vi "Login.vi"(8 "error in (no error)":errorcluster, 11 "reference in":refnum<class "Test_Base.lvclass">) -> (0 "error out":errorcluster, 1 "cancelled":bool, 2 "valid":bool, 3 "reference in":refnum<class "Test_Base.lvclass">)   [LabVIEW 2022 SP3, in "Test_Base.lvlib" / "Test_Base.lvclass"]
uses:
  Test_Base.lvclass
  Components/MES_Base.lvlibp/MES_Base.lvclass
  Components/TestView_Base.lvlibp/TestView_Base.lvclass
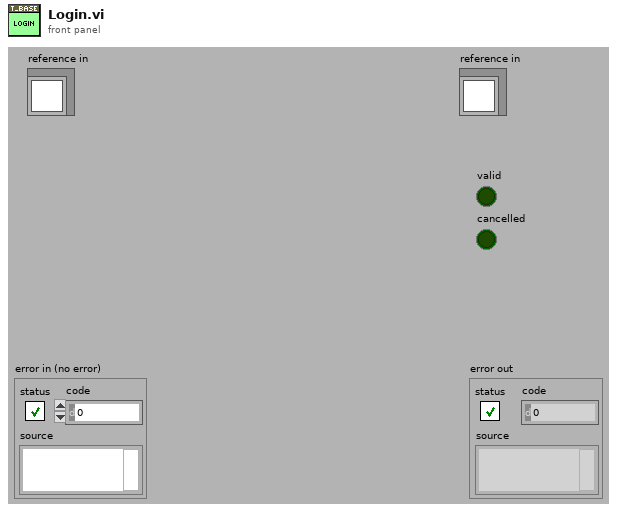
[diagram p1: front panel]
types:
  T1 = typedef "Test_Base.lvlib/Test_Base.lvclass/ObjectAttributes.ctl" = cluster{"Config":T2, "UUTIndex":i32, "Serial":string, "Batch":string, "MES":refnum<class "MES_Base.lvclass">, "TestView":refnum<class "TestView_Base.lvclass">, "LoggedIn":bool, "Abort":bool}
  T2 = typedef "Test_Base.lvlib/Test_Base.lvclass/Config.ctl" = cluster{"ContinueOnFail":bool}
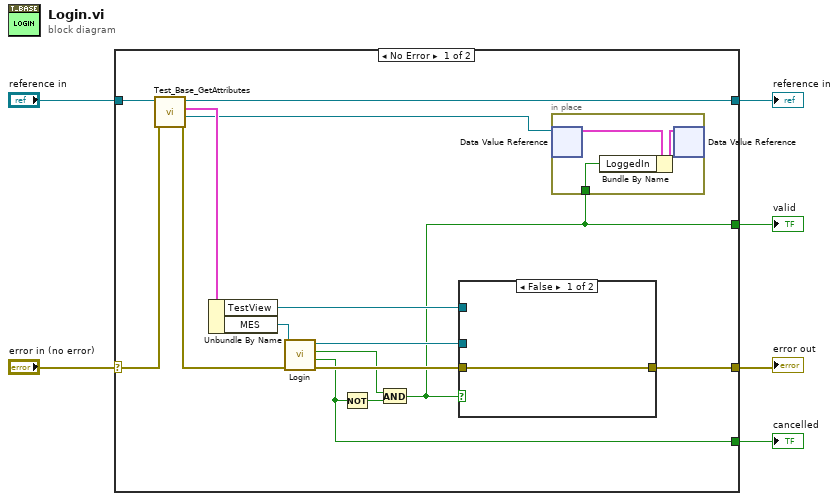
[diagram p0: block diagram]
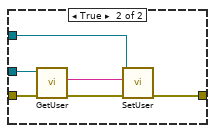
[diagram p2: hidden frame]
diagram:
  n1 = case shown="No Error" "error in (no error)" {
    selector: "error in (no error)" -> [w21 w33]
    tunnel: [w13 w33] -> w5
    tunnel: [w18 w32] -> w3
    tunnel: "reference in" -> [w19 w32]
    tunnel: [w9 _] -> w2
    tunnel: [w7 _] -> w1
    frame No Error {
      n2 = call "Test_Base_GetAttributes.vi"("error in (no error)"=w21, "reference in"=w19) -> ("error out"=w16:errorcluster, "DataRef"=w15:refnum<data-value>, "Data"=w20:T1, "reference out"=w18:refnum<class "Test_Base.lvclass">)  [unwired: 6 in]
      n3 = Unbundle By Name(w20) -> ("TestView"=w11:refnum<class "TestView_Base.lvclass">, "MES"=w17:refnum<class "MES_Base.lvclass">)
      n4 = call-dynamic "Login.vi"("error in (no error)"=w16, "reference in"=w17) -> ("error out"=w14:errorcluster, "Cancelled"=w7:bool, "Valid"=w10:bool, "reference in"=w12:refnum<class "MES_Base.lvclass">)  [unwired: 5 in]
      n5 = Not(x=w7) -> (.not. x?=w8:bool)
      n6 = And(x=w10, y=w8) -> (x .and. y?=w9:bool)
      n7 = case shown="False" w9 {
        tunnel: w14 -> [w22 w28]
        tunnel: [w22 w25] -> w13
        tunnel: w12 -> [_ w27]
        tunnel: w11 -> [_ w24]
        frame False {
        }
        frame True {
          n8 = call-dynamic "GetUser.vi"("error in (no error)"=w28, "reference in"=w27) -> ("error out"=w26:errorcluster, "User"=w23:string)  [unwired: 6 in, 2 out]
          n9 = call-dynamic "SetUser.vi"("error in (no error)"=w26, "User"=w23, "reference in"=w24) -> ("error out"=w25:errorcluster)  [unwired: 7 in, 1 out]
        }
      }
      n10 = in-place {
        in-place-border: w9 -> [w29]
        n11 = in-place-dvr #1(w15) -> (w31:T1)  [unwired: 1 out]
        n12 = Bundle By Name(cluster=w31, "LoggedIn"=w29) -> (w30:T1)
        n13 = in-place-dvr #1(w30) -> ()  [unwired: 2 out]
      }
    }
    frame Error {
    }
  }
  "error out" <- w5
  "reference in" <- w3
  "valid" <- w2
  "cancelled" <- w1
